vi "find_best_phase.vi"(8 "steepest slope":dbl, 9 "phase in":dbl, 10 "steepest slope array in":dbl[](array[numeric]), 11 "index":i32) -> (1 "complete":bool, 2 "optimum phase":dbl, 3 "steepest slope array out":dbl[](array[numeric]))   [LabVIEW 2015]
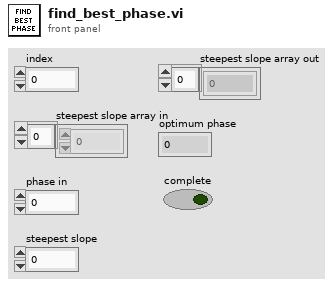
[diagram p1: front panel]
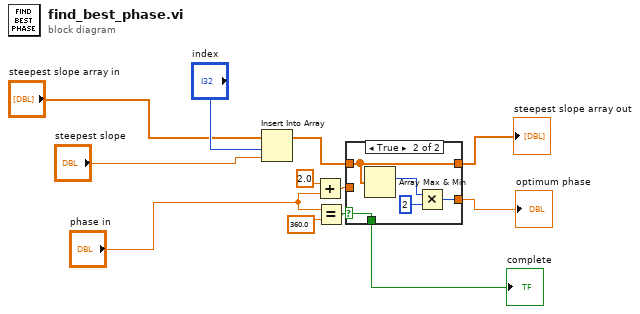
[diagram p0: block diagram]
diagram:
  n1 = Insert Into Array(array="steepest slope array in", index="index", new element="steepest slope") -> (w9:dbl[])
  n2 = Add(x=2.0 ("y"), y="phase in") -> (x+y=w10:dbl)
  n3 = Equal?(x="phase in", y=360.0) -> (x = y?=w8:bool)
  n4 = case shown="True" w8 {
    selector: w8 -> [w13 w17]
    tunnel: w9 -> [w15 w18]
    tunnel: [w15 w18] -> w4
    tunnel: w10 -> [w14 _]
    tunnel: [w14 w19] -> w2
    tunnel: [w13 w17] -> w6
    frame False {
    }
    frame True {
      n5 = Array Max & Min(array=w18) -> (max index (indices)=w16:i32)  [unwired: 3 out]
      n6 = Multiply(x=w16, y=2) -> (x*y=w19:i32)
    }
  }
  "complete" <- w6
  "steepest slope array out" <- w4
  "optimum phase" <- w2
